vi "_Destroy.vi"(8 "error in (no error)":errorcluster, 11 "Temperature Control in":refnum<class "Temperature Control.lvclass">) -> (0 "error out":errorcluster, 2 "Finalized Readable":refnum<class "Readable.lvclass">)   [LabVIEW 2009, in "Temperature Control.lvclass"]
doc: "Release resources from and deallocate this Reader instance."
uses:
  Temperature Control.lvclass
  Reader/Reader.lvclass
  Instruments/Utility Classes/Readable/Readable.lvclass
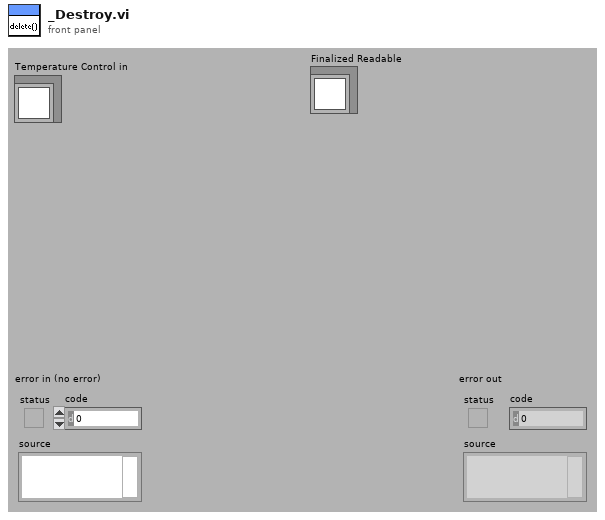
[diagram p1: front panel]
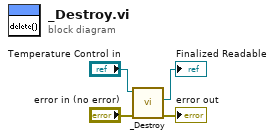
[diagram p0: block diagram]
diagram:
  n1 = call-parent "_Destroy.vi"("error in (no error)"="error in (no error)", "Reader in"="Temperature Control in") -> ("error out"=→"error out":errorcluster, "Finalized Readable"=→"Finalized Readable":refnum<class "Readable.lvclass">)  [unwired: 8 in]
